vi "Replace Missing Dependency VIs - Client Wrapper.vi"(8 "error in":errorcluster, 9 "New Subname":string, 10 "Proto Names":T1, 11 "Template Project Path":path) -> (0 "error out":errorcluster)   [LabVIEW 2021, in "Plugin Generator.lvlib"]
uses:
  Plugin Generator.lvlib
  Typedef/Proto Names.ctl
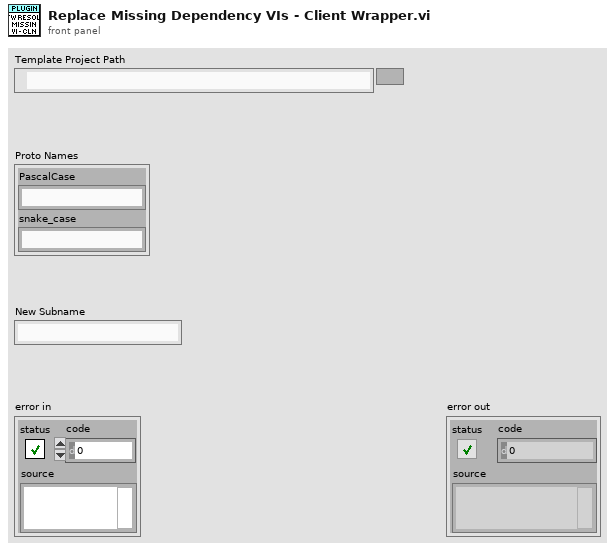
[diagram p1: front panel]
types:
  T1 = typedef "Plugin Generator.lvlib/Proto Names.ctl" = cluster{"PascalCase":string, "snake_case":string}
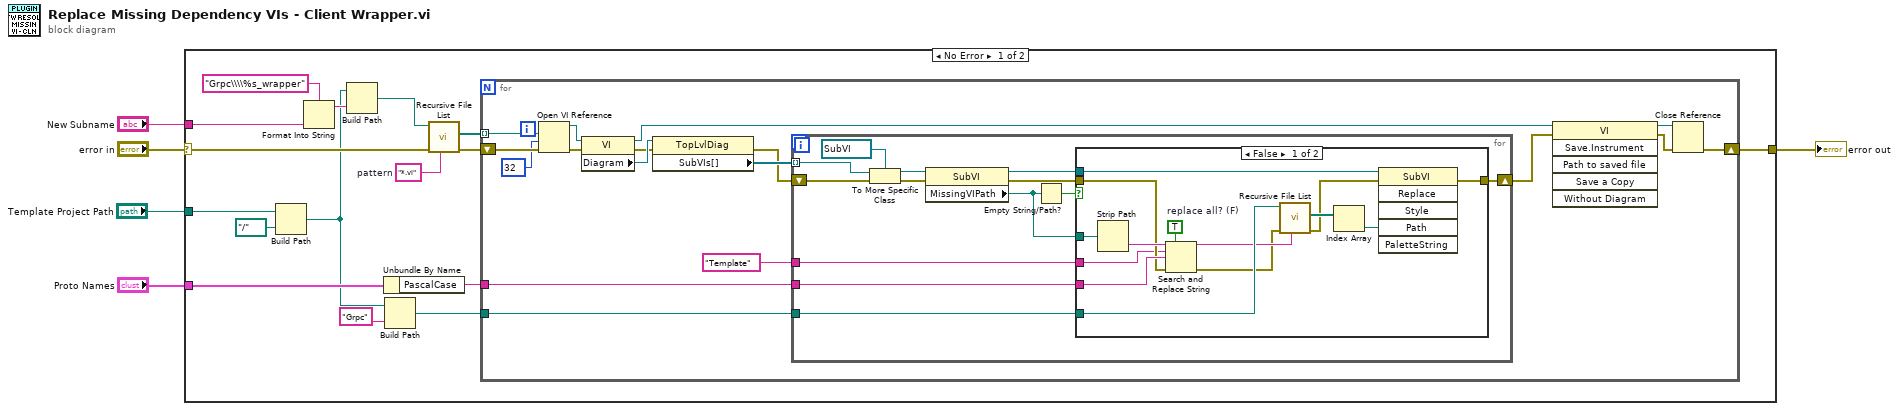
[diagram p0: block diagram]
diagram:
  n1 = case shown="No Error" "error in" {
    selector: "error in" -> [w16 w67]
    tunnel: [w15 w67] -> w5
    tunnel: "Template Project Path" -> [w13 _]
    tunnel: "New Subname" -> [w11 _]
    tunnel: "Proto Names" -> [w10 _]
    frame No Error {
      w20 = "*.vi"  # pattern
      n2 = Build Path(base path=w13, name or relative path=path "../..") -> (appended path=w8:path)
      n3 = Format Into String(format string="Grpc\\\\%s_wrapper" ("Class Name"), w11) -> (resulting string=w19:string)  [unwired: 2 in, 1 out]
      n4 = Build Path(base path=w8, name or relative path=w19) -> (appended path=w12:path)
      n5 = Unbundle By Name(w10) -> ("PascalCase"=w9:string)
      n6 = Build Path(base path=w8, name or relative path="Grpc" ("Class Name")) -> (appended path=w6:path)
      n7 = call <vilib>:"Recursive File List.vi"("pattern"=w20, "error in (no error)"=w16, "Folder Path"=w12) -> ("error out"=w17:errorcluster, "All Files in Dir"=w21:path[])  [unwired: 4 in, 3 out]
      n8 = for {
        tunnel: w21 -> [w38] mode=indexing
        tunnel: w9 -> [w37]
        shift-right: [w36] -> w15
        shift-left: w17 -> [w35]
        tunnel: w6 -> [w22]
        n9 = Open VI Reference(vi path=w38, options=32, error in (no error)=w35) -> (vi reference=w34:refnum<vi>, error out=w29:errorcluster)  [unwired: 3 in]
        n10 = property class="VI"(reference=w34, error in=w29) -> (reference out=w32:refnum<vi>, error out=w30:errorcluster, "Diagram"=w33:refnum<vi>)
        n11 = property class="TopLvlDiag"(reference=w33, error in=w30) -> (error out=w24:errorcluster, "SubVIs[]"=w31:refnum<vi>[])  [unwired: 1 out]
        n12 = for {
          tunnel: w31 -> [w51] mode=indexing
          tunnel: w37 -> [w49]
          tunnel: "Template" ("search string") -> [w39]
          shift-right: [w50] -> w23
          shift-left: w24 -> [w48]
          tunnel: w22 -> [w47]
          n13 = To More Specific Class(target class=refnum<vi> refnum ("x"), reference=w51, error in=w48) -> (specific class reference=w41:refnum<vi>, error out=w40:errorcluster)
          n14 = property class="SubVI"(reference=w41, error in=w40) -> (reference out=w45:refnum<vi>, error out=w43:errorcluster, "MissingVIPath"=w44:path)
          n15 = Empty String/Path?(string/path=w44) -> (empty?=w46:bool)
          n16 = case shown="False" w46 {
            tunnel: w45 -> [w65 _]
            tunnel: w44 -> [w57 _]
            tunnel: w49 -> [w64 _]
            tunnel: w43 -> [w54 w66]
            tunnel: [w62 w66] -> w50
            tunnel: w47 -> [w58 _]
            tunnel: w39 -> [w52 _]
            frame False {
              w63 = TRUE  # replace all? (F)
              n17 = Strip Path(path=w57) -> (name=w56:string)  [unwired: 1 out]
              n18 = Search and Replace String(replace all?=w63, input string=w56, search string=w52, replace string=w64, error in=w54) -> (result string=w55:string, error out=w53:errorcluster)  [unwired: 3 in, 2 out]
              n19 = call <vilib>:"Recursive File List.vi"("pattern"=w55, "error in (no error)"=w53, "Folder Path"=w58) -> ("error out"=w59:errorcluster, "All Files in Dir"=w61:path[])  [unwired: 4 in, 3 out]
              n20 = Index Array(array=w61) -> (element=w60:path)  [unwired: 1 in]
              n21 = invoke class="SubVI" method="Replace"(reference=w65, error in=w59, "Path"=w60) -> (error out=w62:errorcluster)  [unwired: 3 in, 5 out]
            }
            frame True {
            }
          }
        }
        n22 = invoke class="VI" method="Save.Instrument"(reference=w32, error in=w23) -> (reference out=w27:refnum<vi>, error out=w26:errorcluster)  [unwired: 4 in, 4 out]
        n23 = Close Reference(reference=w27, error in (no error)=w26) -> (error out=w36:errorcluster)
      }
    }
    frame Error {
    }
  }
  "error out" <- w5
